vi "niDTS Template RF Test Configure.vi"(0 "Template Tx Test Handle in":T2, 7 "Parameters":T1, 9 "ResultsIndex":u8=1, 11 "error in (no error)":errorcluster) -> (4 "Template Tx Test Handle out":T2, 15 "error out":errorcluster)   [LabVIEW 2014, in "niDTS Template.lvlib"]
uses:
  niDTS Template.lvlib
  Includes/Template RF Test INC Handle.ctl
  Objects/BASE_class/Template RF Test.lvclass
  Includes/Template RF Test INC Parameters.ctl
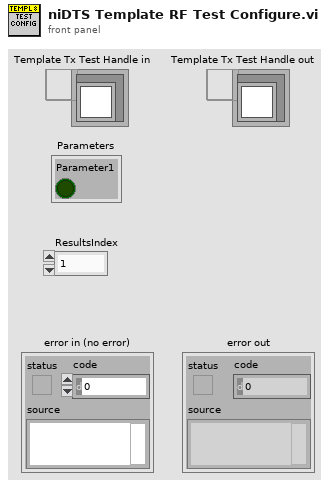
[diagram p1: front panel]
types:
  T1 = typedef "niDTS Template.lvlib/Template RF Test INC Parameters.ctl" = cluster{"Parameter1":bool}
  T2 = typedef "niDTS Template.lvlib/Template RF Test INC Handle.ctl" = refnum<data-value>
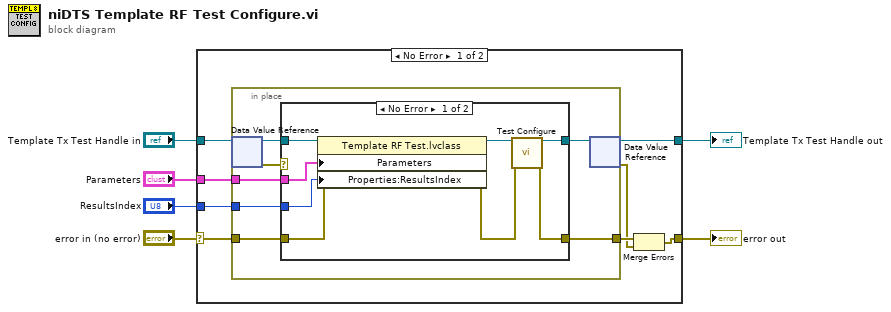
[diagram p0: block diagram]
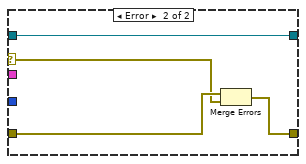
[diagram p2: hidden frame]
diagram:
  n1 = case shown="No Error" "error in (no error)" {
    selector: "error in (no error)" -> [w10 w34]
    tunnel: "Parameters" -> [w14 _]
    tunnel: "Template Tx Test Handle in" -> [w13 w35]
    tunnel: [w12 w35] -> w4
    tunnel: [w8 w34] -> w3
    tunnel: "ResultsIndex" -> [w11 _]
    frame No Error {
      n2 = in-place {
        in-place-border: w10 -> [w18]
        in-place-border: [w17] -> w9
        in-place-border: w14 -> [w16]
        in-place-border: w11 -> [w15]
        n3 = in-place-dvr #1(w13) -> (w20:refnum<class "Template RF Test.lvclass">, w21:errorcluster)
        n4 = case shown="No Error" w21 {
          selector: w21 -> [_ w31]
          tunnel: w20 -> [w29 w33]
          tunnel: [w25 w33] -> w19
          tunnel: w18 -> [w28 w32]
          tunnel: [w26 w30] -> w17
          tunnel: w16 -> [w23 _]
          tunnel: w15 -> [w22 _]
          frame No Error {
            n5 = property class="Template RF Test.lvclass"(reference=w29, error in=w28, "Parameters"=w23, "Properties:ResultsIndex"=w22) -> (reference out=w24:refnum<class "Template RF Test.lvclass">, error out=w27:errorcluster)
            n6 = call-dynamic "Test Configure.vi"("Template Tx Test in"=w24, "error in (no error)"=w27) -> ("Template Tx Test out"=w25:refnum<class "Template RF Test.lvclass">, "error out"=w26:errorcluster)  [unwired: 12 in]
          }
          frame Error {
            n7 = Merge Errors(w32, w31) -> (w30:errorcluster)
          }
        }
        n8 = in-place-dvr #1(w19) -> (w12:T2, w7:errorcluster)
      }
      n9 = Merge Errors(w9, w7) -> (w8:errorcluster)
    }
    frame Error {
    }
  }
  "Template Tx Test Handle out" <- w4
  "error out" <- w3
